vi "Agilent3446X_Init.vi"(8 "error in":errorcluster caption="错误输入", 11 "MyIndex":u8) -> (0 "error out":errorcluster caption="错误输出", 3 "OK?":bool)   [LabVIEW 2015]
uses:
  Agilent 3446X Series/Agilent 3446X Series1.lvlib
panel:
  out "read buffer":string
  out "VISA resource out":refnum<visa-resource-name>
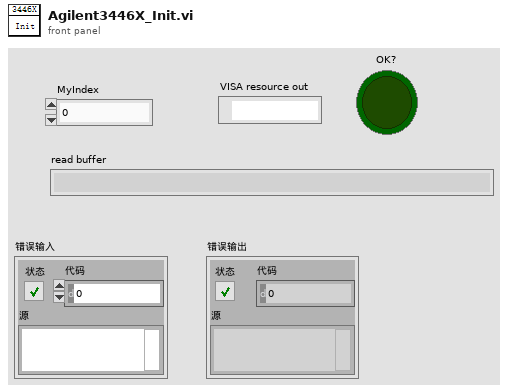
[diagram p1: front panel]
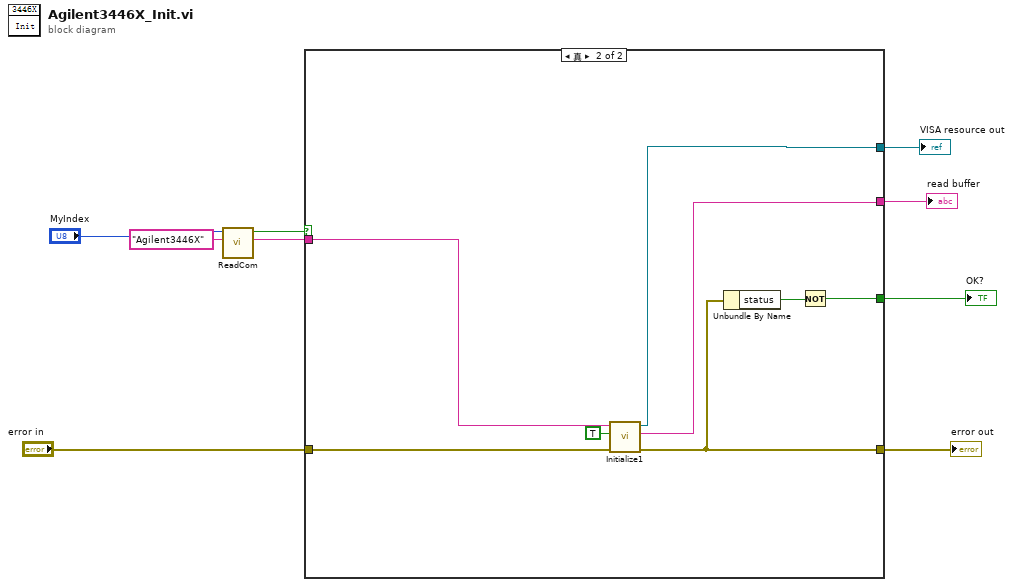
[diagram p0: block diagram]
diagram:
  n1 = call "ReadCom.vi"("仪器名称"="Agilent3446X", "MyIndex"="MyIndex") -> ("COM"=w2:string, "OK?"=w4:bool)  [unwired: 7 in, 1 out]
  n2 = case shown="真" w4 {
    tunnel: [_ w12] -> w9
    tunnel: [_ w17] -> w8
    tunnel: [_ w16] -> w7
    tunnel: "error in" -> [_ w14]
    tunnel: w2 -> [_ w13]
    tunnel: [_ w10] -> w1
    frame False {
    }
    frame True {
      n3 = call "Initialize1.vi"("error in (no error)"=w14, "ID Query (True)"=TRUE, "VISA resource name"=w13) -> ("error out"=w12:errorcluster, "read buffer"=w16:string, "VISA resource name out"=w17:refnum<visa-resource-name>)  [unwired: 2 in, 4 out]
      n4 = Unbundle By Name(w12) -> ("status"=w11:bool)
      n5 = Not(x=w11) -> (.not. x?=w10:bool)
    }
  }
  "error out" <- w9
  "VISA resource out" <- w8
  "read buffer" <- w7
  "OK?" <- w1
